vi "Main.vi"() -> ()   [LabVIEW 2020]
uses:
  Controls/Pages.ctl
  Controls/ManualTestParameters.ctl
  Controls/AutomaticalTestParameters.ctl
  <vilib>/express/express analysis/Spectral/Block/exnSpectralBlock spectral measurements power poly.vi
  <vilib>/express/express analysis/Spectral/Block/exnSpectralBlock spectral measurements power DDT.vi
  <vilib>/Utility/file.llb/Write Delimited Spreadsheet (string).vi
  <vilib>/express/express analysis/Spectral/XNode/ExpressSpectralMeasurementsBlockNode.xnode
panel:
  in  "Tab Control":T1=enum."自動測試/Automatical Test"
  in  "Manual Stop":bool
  in  "Manual Start":bool
  out "REVO. Alternate":dbl
  out "Manual Deflection":dbl
  out "BEND. Moment":dbl
  out "Tachometer":dbl
  in  "Order Open":bool
  in  "Auto Open":bool
  in  "Drive Up":bool
  in  "Drive Down":bool
  in  "Lamp On":bool
  in  "Lamp Off":bool
  out "Deflection":cluster{"probe x":dbl[], "probe y":dbl[]}[](graph)
  out "Power Spectrum":dynamicdata(graph)=[{"t0"=timestamp(0 s since 1904-01-01), "dt"=10.0, "Y"=[7.532951334960212e-36, 1.7210013073600366e-33, 2.9039505459542225e-32, 9.336804130865817e-32, 3.125000000000003, 12.499999999999991, 3.1249999999999942, 1.4832349234044934e-31, 1.9137290229811662e-32, 1.276010813808381e-32, 1.540768629947705e-33, 7.89098636152294e-33, 3.719445115484756e-33, 2.1300708903905205e-33, 4.0510738555792935e-32, 4.175831739872474e-32, 7.199150609282058e-32, 7.992518441924071e-34, 3.15189982829308e-33, 1.5483081913227212e-32, 1.6373277826284248e-32, 2.2138266275822093e-34, 4.406252635318449e-33, 3.438771975347449e-33, 1.3240311408006708e-32, 1.864729947416446e-31, 3.1076446481504366e-32, 1.351580401177905e-32, 1.0666709108251642e-32, 3.703047405966511e-33, 6.290037498430406e-32, 1.2794414884957584e-33, 3.841586151461403e-33, 7.984806335457992e-34, 3.5638767150319115e-32, 4.1301066800437274e-32, 4.0393850154926674e-32, 3.13032293215036e-33, 1.4282906971287278e-33, 3.758265447602662e-33, 1.0313371534831396e-31, 1.0624643515683048e-32, 4.981671705505977e-33, 1.9271055708889898e-33, 3.687743394522952e-32, 2.70478781889346e-31, 6.205033963623051e-32, 3.6208769442789164e-32, 9.98040293718275e-33, 2.859575628363253e-33], "attributes"=variant("NI_ChannelName"=variant(string "Sine (Power Spectrum)"), "NI_ExpIsRelativeTime"=variant(bool TRUE), "NI_ExpStartTimeStamp"=variant(timestamp timestamp(3762475107.3663697 s since 1904-01-01)), "NI_ExpTimeStamp"=variant(timestamp timestamp(3762475118.76637 s since 1904-01-01)), "NI_ExpXDimension"=variant(string "f"), "NI_OriginalChannelName"=variant(string "Sine"))}]
  in  "Reso Start":bool
  in  "Reso Stop":bool
  out "EstimatedTime_Value":dbl=290.99090337753296 format="%#_3g"
  in  "Auto Stop":bool
  out "Deflection_Value":dbl
  in  "Deflection_Setting":dbl=0.8
  out "Cycles_Value":dbl
  in  "Cycles_Setting":dbl=100.0
  out "BEND. Moment_Value":dbl
  in  "BEND. Moment_Setting":dbl=95.0
  out "Tachometer_Value":dbl
  in  "Tachometer_Setting":dbl=200.0
  out "Machine STA.":string="Running"
  in  "Auto Start":bool
  in  "Table":string[][](table)
  in  "Save Button":bool
  # "輪圈彎曲力矩耐久測試機"
  # "CORNERING BENDING ENDURANCE TESTER"
  # "金嵩盛機械股份有限公司承製"
  # "King Swen Sheng Machinery Co, Ltd."
  # "FAX: 886-3-4561597"
  # "TEL: 886-3-4384699"
  # "手動測試"
  # "Manual Test"
  # "迴轉轉速/Tachometer:"
  # "RPM"
  # "彎曲力矩/BEND. Moment:"
  # "N．m"
  # "負載偏移量/Deflection:"
  # "mm"
  # "主軸間距/REVO. Alternate:"
  # "M/M"
  # "共振測試"
  # "Resonance Test"
  # "自動測試"
  # "Automatical Test"
  # "機台狀況/Machine STA. :"
  # "設定值/Setting"
  # "實際值/Value"
  # "迴轉轉速/Tachometer:"
  # "RPM"
  # "力矩/BEND. Moment:"
  # "N．m"
  # "圈數/INT. Cycles:"
  # "圈"
  # "偏移量/Deflection:"
  # "mm"
  # "預計完成時間/Estimated Finish Time:"
  # "mins"
  # "報告產生"
  # "Report Generation"
  # "輪圈彎曲力矩耐久測試機"
  # "CORNERING BENDING ENDURANCE TESTER"
  # "金嵩盛機械股份有限公司承製"
  # "King Swen Sheng Machinery Co, Ltd."
  # "FAX: 886-3-4561597"
  # "TEL: 886-3-4384699"
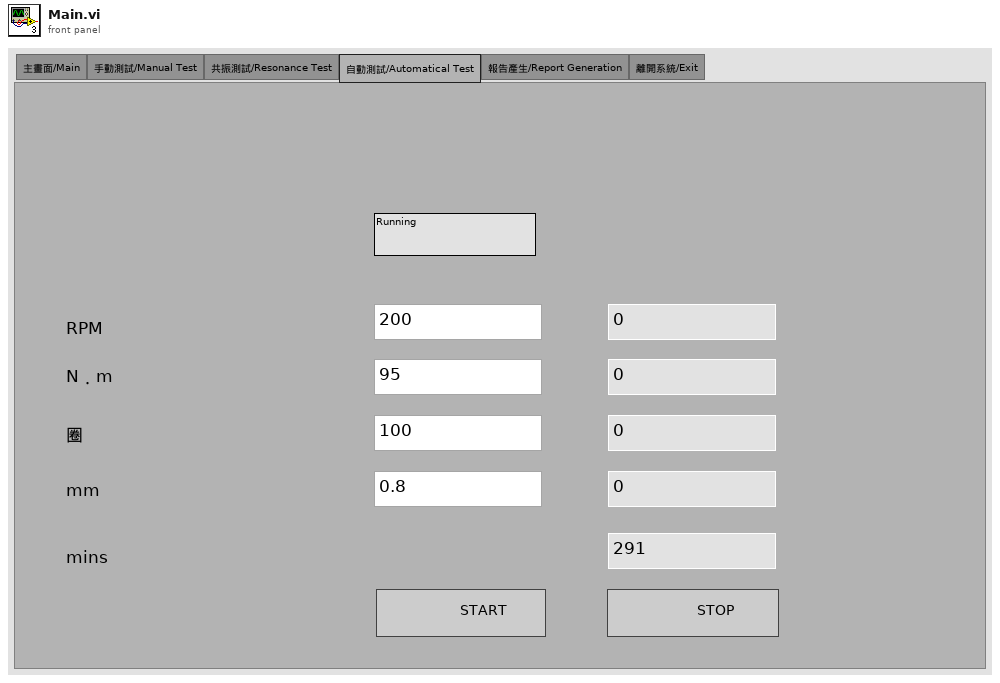
[diagram p1: front panel]
types:
  T1 = typedef "Pages.ctl" = enum32{"主畫面/Main", "手動測試/Manual Test", "共振測試/Resonance Test", "自動測試/Automatical Test", "報告產生/Report Generation", "離開系統/Exit"}
  T2 = typedef "AutomaticalTestParameters.ctl" = cluster{"Machine STA.":string, "Tachometer_Setting":dbl, "BEND. Moment_Setting":dbl, "Cycles_Setting":dbl, "Deflection_Setting":dbl, "Tachometer_Value":dbl, "BEND. Moment_Value":dbl, "Cycles_Value":dbl, "Deflection_Value":dbl, "EstimatedTime_Value":dbl, "Play Button":bool, "Stop Button":bool}
  T3 = typedef "ManualTestParameters.ctl" = cluster{"Order Open":bool, "Auto Open":bool, "Drive Up":bool, "Drive Down":bool, "Lamp On":bool, "Lamp Off":bool, "Tachometer":dbl, "BEND. Moment":dbl, "Deflection":dbl, "REVO. Alternate":dbl, "Drive Up Limit":dbl}
  T4 = enum8{"Enabled", "Disabled", "Disabled and Grayed Out"}
  T5 = cluster{"averaging mode":u16, "weighting mode":u16, "number of averages":u32}
  T6 = cluster{"dB On (F)":bool, "unwrap phase (F)":bool, "convert to degree (F)":bool}
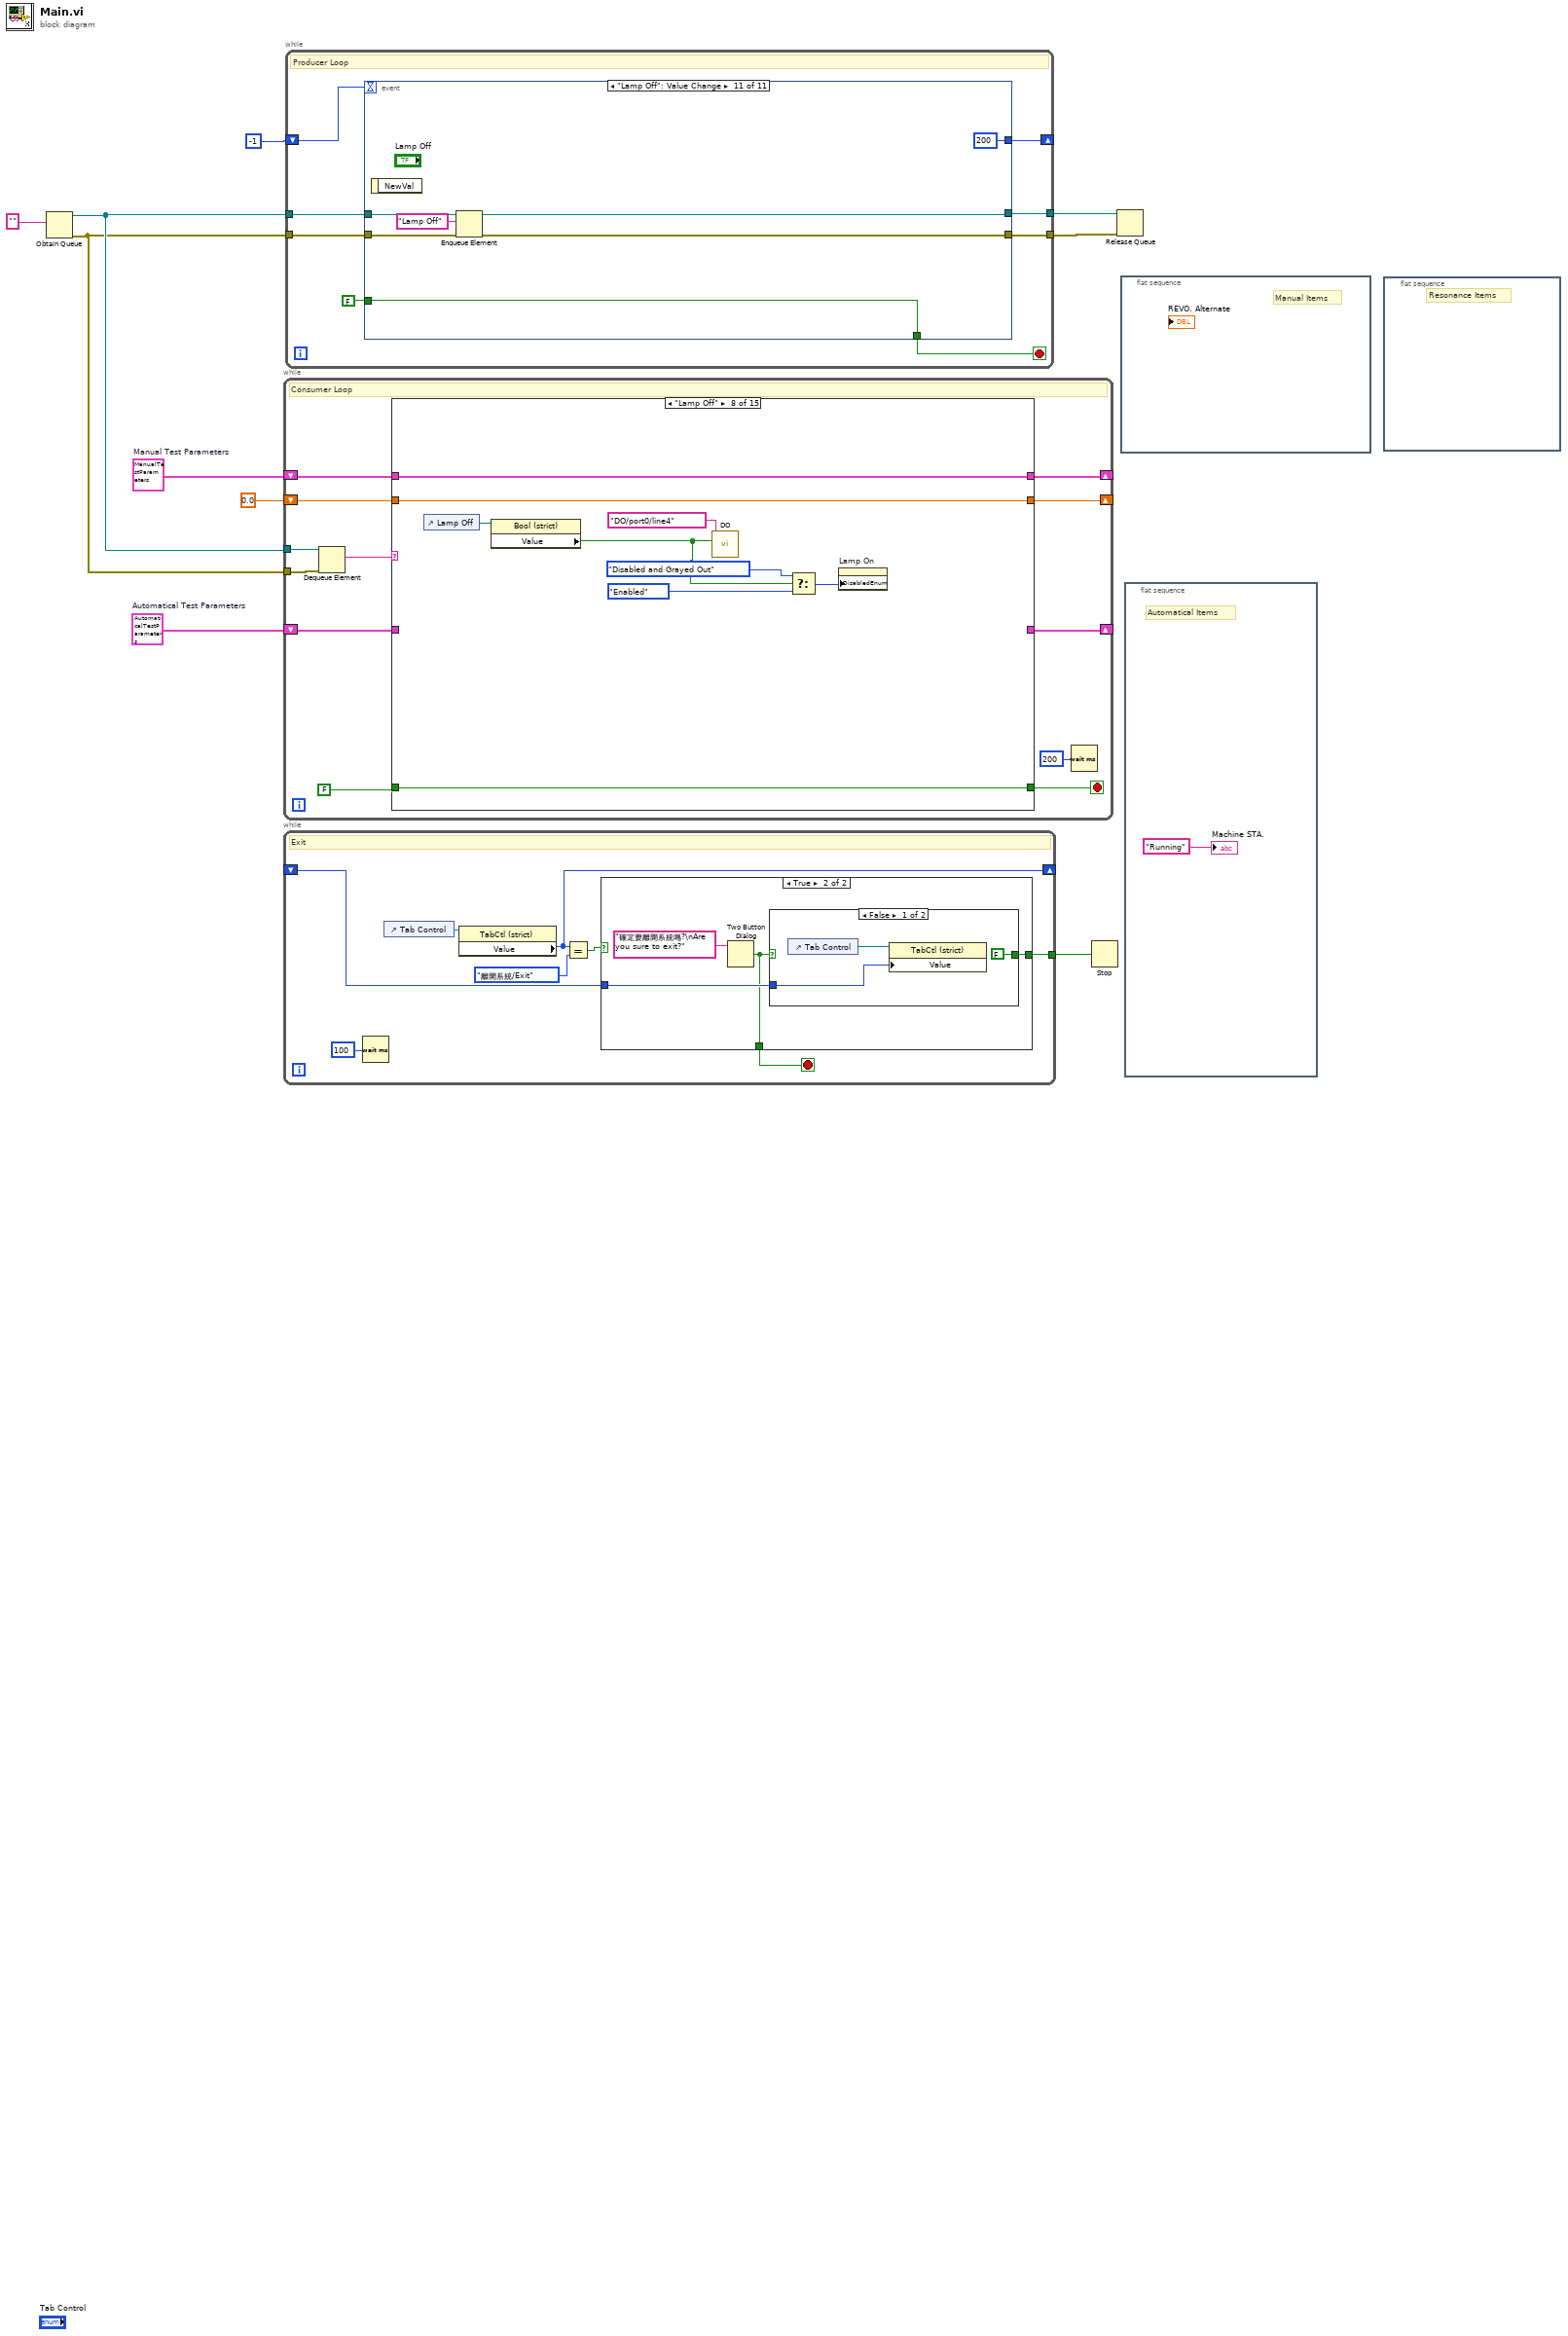
[diagram p0: block diagram]
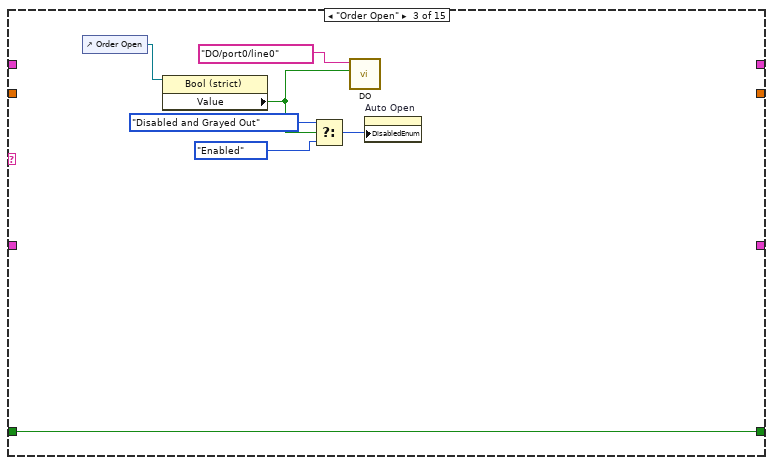
[diagram p4: hidden frame]
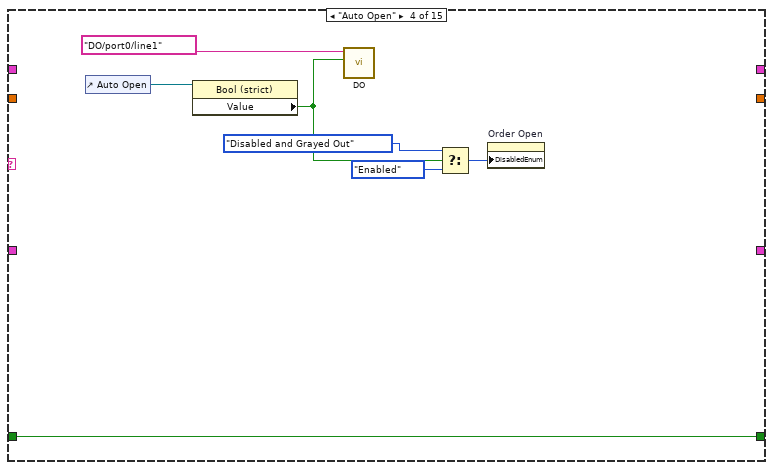
[diagram p5: hidden frame]
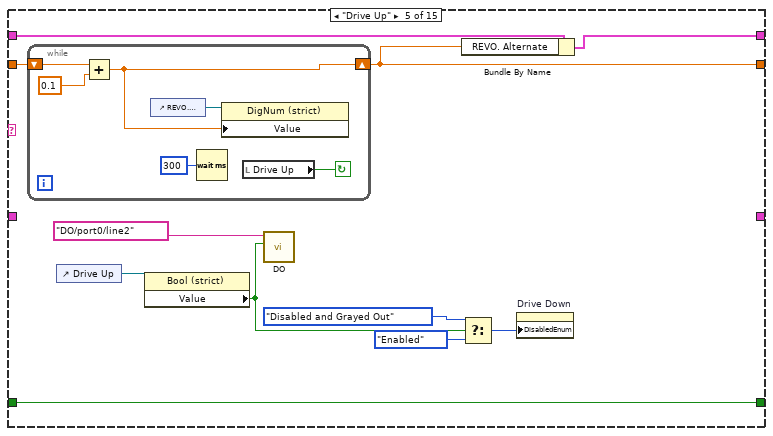
[diagram p6: hidden frame]
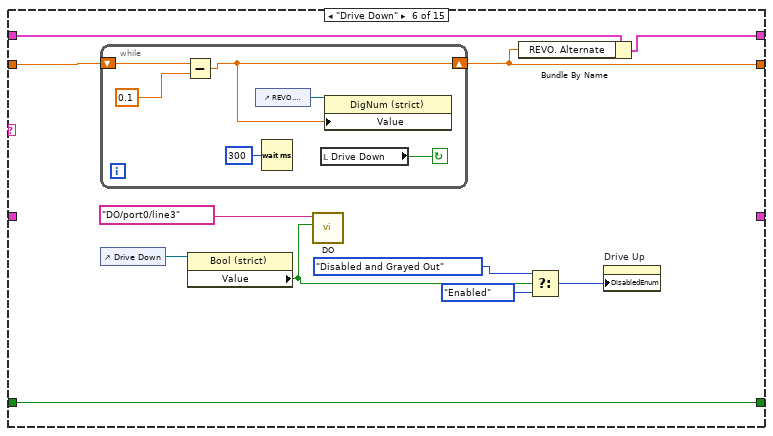
[diagram p7: hidden frame]
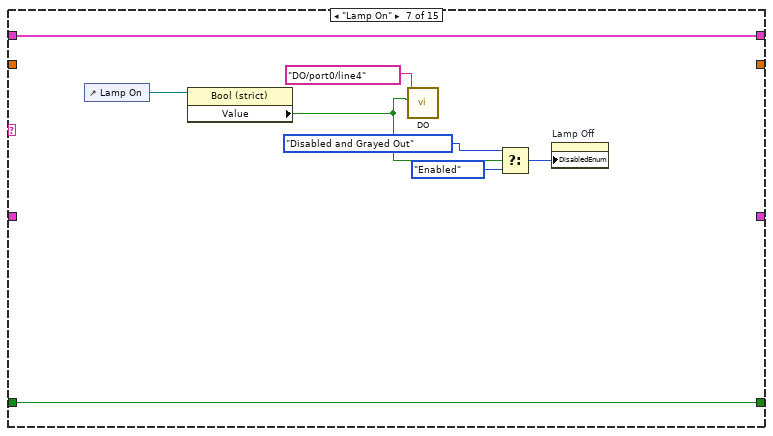
[diagram p8: hidden frame]
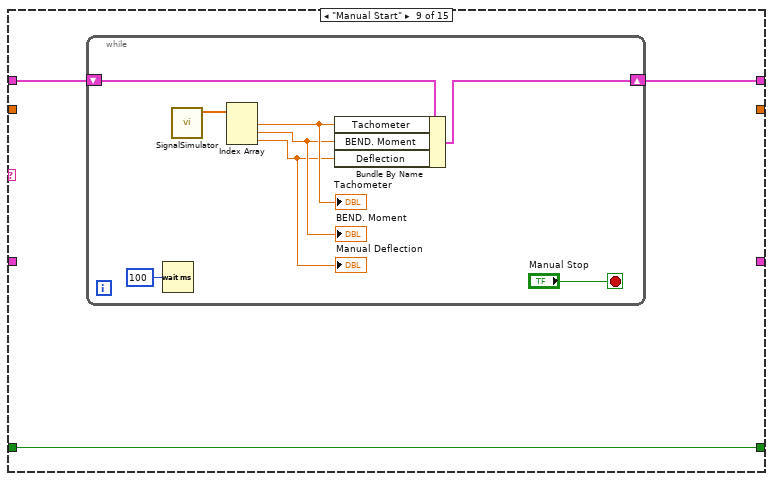
[diagram p9: hidden frame]
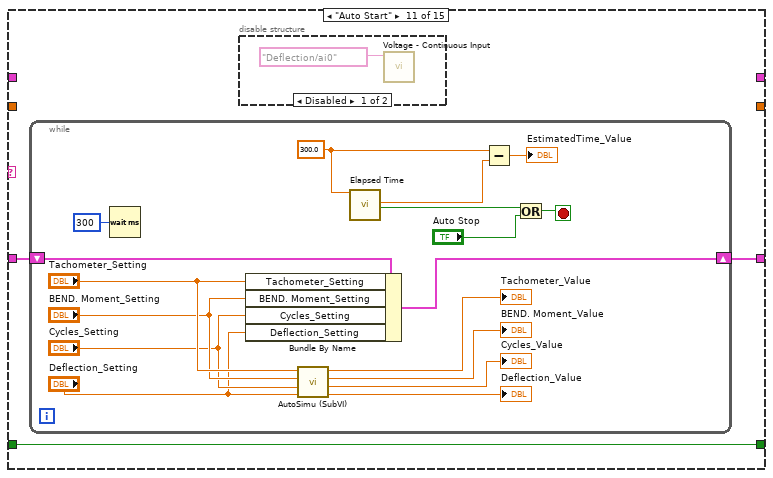
[diagram p11: hidden frame]
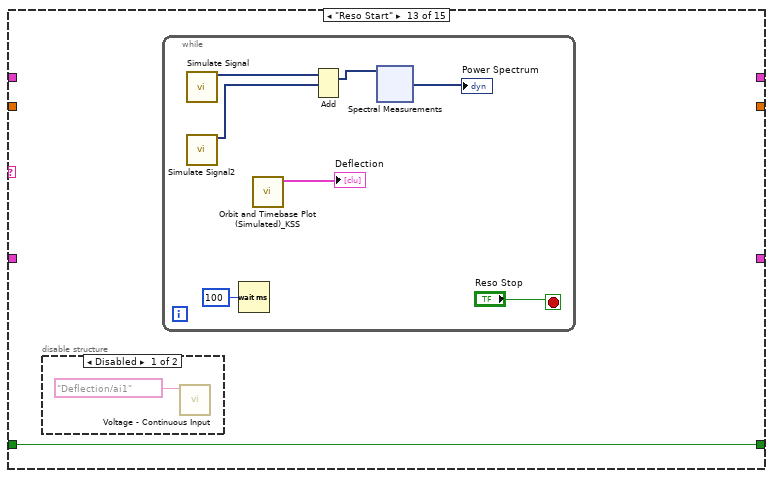
[diagram p14: hidden frame]
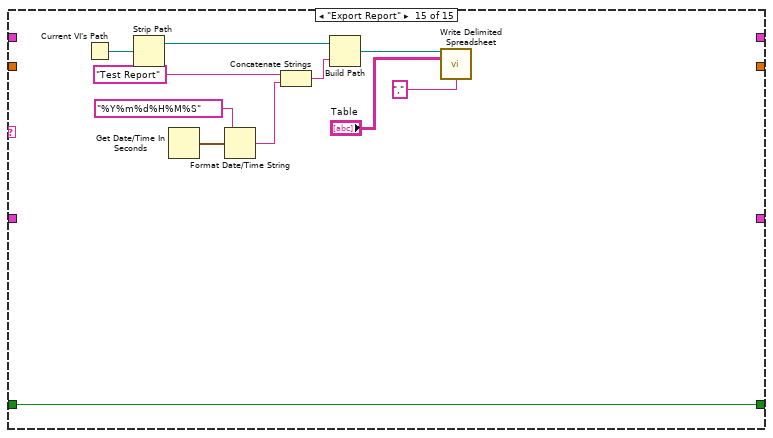
[diagram p17: hidden frame]
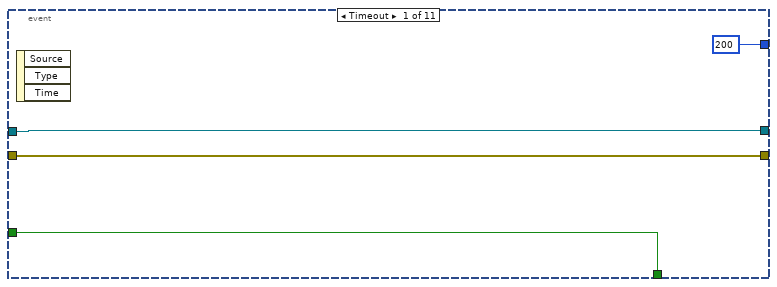
[diagram p18: hidden frame]
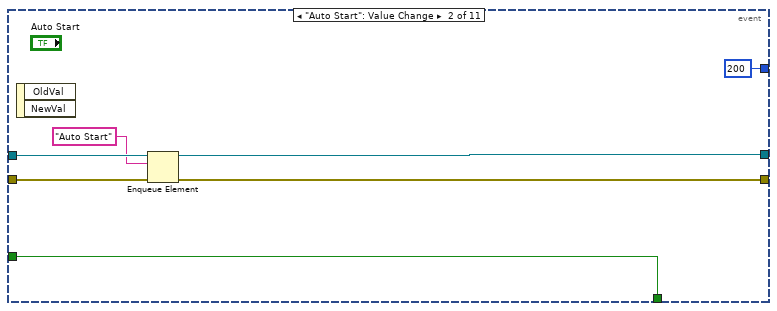
[diagram p19: hidden frame]
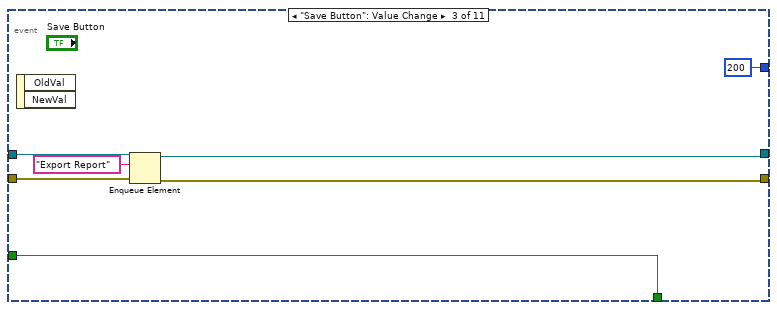
[diagram p20: hidden frame]
diagram:
  w1 = T2 {"Machine STA."="", "Tachometer_Setting"=0.0, "BEND. Moment_Setting"=0.0, "Cycles_Setting"=0.0, "Deflection_Setting"=0.0, "Tachometer_Value"=0.0, "BEND. Moment_Value"=0.0, "Cycles_Value"=0.0, "Deflection_Value"=0.0, "EstimatedTime_Value"=0.0, "Play Button"=FALSE, "Stop Button"=FALSE}  # Automatical Test Parameters
  w3 = T3 {"Order Open"=FALSE, "Auto Open"=FALSE, "Drive Up"=FALSE, "Drive Down"=FALSE, "Lamp On"=FALSE, "Lamp Off"=FALSE, "Tachometer"=0.0, "BEND. Moment"=0.0, "Deflection"=0.0, "REVO. Alternate"=0.0, "Drive Up Limit"=0.0}  # Manual Test Parameters
  n1 = Obtain Queue(element data type="") -> (queue out=w8:refnum<queue>, error out=w7:errorcluster)  [unwired: 4 in, 1 out]
  n2 = while {
    tunnel: w8 -> [w22]
    tunnel: w7 -> [w21]
    shift-right: [w16] -> _
    shift-left: w3 -> [w17]
    shift-right: [w14] -> _
    shift-left: 0.0 -> [w15]
    shift-right: [w11] -> _
    shift-left: w1 -> [w12]
    stop <- w19 stop-if-true
    # "Consumer Loop"
    n3 = Dequeue Element(queue=w22, error in (no error)=w21) -> (element=w20:string)  [unwired: 1 in, 3 out]
    n4 = case shown="\"Lamp Off\"" w20 {
      tunnel: [w23 w24 w31 w38 w49 w66 w80 w89 w92 w103 w106 w125 w126 w144 w155] -> w19
      tunnel: FALSE -> [w23 w24 w31 w38 w49 w66 w80 w89 w92 w103 w106 w125 w126 w144 w155]
      tunnel: w17 -> [_ _ _ _ w46 w63 w78 w87 w91 w102 _ _ _ _ _]
      tunnel: [_ _ _ _ w44 w62 w78 w87 w90 w102 _ _ _ _ _] -> w16
      tunnel: w15 -> [_ _ _ _ w45 w61 _ w86 _ w101 _ _ _ _ _]
      tunnel: [_ _ _ _ w43 w60 _ w86 _ w101 _ _ _ _ _] -> w14
      tunnel: w12 -> [_ _ _ _ _ _ _ _ _ _ w105 _ _ _ _]
      tunnel: [_ _ _ _ _ _ _ _ _ _ w104 _ _ _ _] -> w11
      frame "False", Default {
      }
      frame "-----Manual Test-----" {
      }
      frame "Order Open" {
        n5 = control-ref of="Order Open"() -> (w29:refnum<vi>)
        n6 = property class="Bool (strict)"(reference=w29) -> ("Value"=w28:bool)  [unwired: 1 in, 2 out]
        n7 = Select(t=T4."Disabled and Grayed Out", s=w28, f=T4."Enabled" ("Disabled")) -> (s? t:f=w25:T4)
        n8 = call "DO.vi"("data"=w28, "Line(s)"=tag "DO/port0/line0") -> ()  [unwired: 9 in, 1 out]
        n9 = property on="Auto Open" class="Bool (strict)"("DisabledEnum"=w25) -> ()  [unwired: 2 in, 2 out]
      }
      frame "Auto Open" {
        n10 = control-ref of="Auto Open"() -> (w36:refnum<vi>)
        n11 = property class="Bool (strict)"(reference=w36) -> ("Value"=w35:bool)  [unwired: 1 in, 2 out]
        n12 = call "DO.vi"("data"=w35, "Line(s)"=tag "DO/port0/line1") -> ()  [unwired: 9 in, 1 out]
        n13 = Select(t=T4."Disabled and Grayed Out" ("Disabled"), s=w35, f=T4."Enabled") -> (s? t:f=w32:T4)
        n14 = property on="Order Open" class="Bool (strict)"("DisabledEnum"=w32) -> ()  [unwired: 2 in, 2 out]
      }
      frame "Drive Up" {
        n15 = while {
          shift-right: [w50] -> w43
          shift-left: w45 -> [w55]
          stop <- w53 continue-if-true
          n16 = Add(x=w55, y=0.1) -> (x+y=w50:dbl)
          n17 = control-ref of="REVO. Alternate"() -> (w51:refnum<vi>)
          n18 = Wait (ms)(milliseconds to wait=u32 300) -> ()  [unwired: 1 out]
          n19 = property class="DigNum (strict)"(reference=w51, "Value"=w50) -> ()  [unwired: 1 in, 2 out]
          n20 = local read "Drive Up"() -> (w53:bool)
        }
        n21 = control-ref of="Drive Up"() -> (w47:refnum<vi>)
        n22 = property class="Bool (strict)"(reference=w47) -> ("Value"=w42:bool)  [unwired: 1 in, 2 out]
        n23 = call "DO.vi"("data"=w42, "Line(s)"=tag "DO/port0/line2") -> ()  [unwired: 9 in, 1 out]
        n24 = Bundle By Name(cluster=w46, "REVO. Alternate"=w43) -> (w44:T3)
        n25 = Select(t=T4."Disabled and Grayed Out" ("Disabled"), s=w42, f=T4."Enabled") -> (s? t:f=w39:T4)
        n26 = property on="Drive Down" class="Bool (strict)"("DisabledEnum"=w39) -> ()  [unwired: 2 in, 2 out]
      }
      frame "Drive Down" {
        n27 = while {
          shift-right: [w69] -> w60
          shift-left: w61 -> [w71]
          stop <- w68 continue-if-true
          n28 = Subtract(x=w71, y=0.1) -> (x-y=w69:dbl)
          n29 = control-ref of="REVO. Alternate"() -> (w70:refnum<vi>)
          n30 = Wait (ms)(milliseconds to wait=u32 300) -> ()  [unwired: 1 out]
          n31 = local read "Drive Down"() -> (w68:bool)
          n32 = property class="DigNum (strict)"(reference=w70, "Value"=w69) -> ()  [unwired: 1 in, 2 out]
        }
        n33 = control-ref of="Drive Down"() -> (w64:refnum<vi>)
        n34 = property class="Bool (strict)"(reference=w64) -> ("Value"=w57:bool)  [unwired: 1 in, 2 out]
        n35 = call "DO.vi"("data"=w57, "Line(s)"=tag "DO/port0/line3") -> ()  [unwired: 9 in, 1 out]
        n36 = Bundle By Name(cluster=w63, "REVO. Alternate"=w60) -> (w62:T3)
        n37 = Select(t=T4."Disabled and Grayed Out" ("Disabled"), s=w57, f=T4."Enabled") -> (s? t:f=w56:T4)
        n38 = property on="Drive Up" class="Bool (strict)"("DisabledEnum"=w56) -> ()  [unwired: 2 in, 2 out]
      }
      frame "Lamp On" {
        n39 = control-ref of="Lamp On"() -> (w74:refnum<vi>)
        n40 = property class="Bool (strict)"(reference=w74) -> ("Value"=w73:bool)  [unwired: 1 in, 2 out]
        n41 = call "DO.vi"("data"=w73, "Line(s)"=tag "DO/port0/line4") -> ()  [unwired: 9 in, 1 out]
        n42 = Select(t=T4."Disabled and Grayed Out" ("Disabled"), s=w73, f=T4."Enabled") -> (s? t:f=w75:T4)
        n43 = property on="Lamp Off" class="Bool (strict)"("DisabledEnum"=w75) -> ()  [unwired: 2 in, 2 out]
      }
      frame "Lamp Off" {
        n44 = control-ref of="Lamp Off"() -> (w82:refnum<vi>)
        n45 = property class="Bool (strict)"(reference=w82) -> ("Value"=w81:bool)  [unwired: 1 in, 2 out]
        n46 = call "DO.vi"("data"=w81, "Line(s)"=tag "DO/port0/line4") -> ()  [unwired: 9 in, 1 out]
        n47 = Select(t=T4."Disabled and Grayed Out" ("Disabled"), s=w81, f=T4."Enabled") -> (s? t:f=w83:T4)
        n48 = property on="Lamp On" class="Bool (strict)"("DisabledEnum"=w83) -> ()  [unwired: 2 in, 2 out]
      }
      frame "Manual Start" {
        n49 = while {
          shift-right: [w96] -> w90
          shift-left: w91 -> [w98]
          stop <- "Manual Stop" stop-if-true
          n50 = Wait (ms)(milliseconds to wait=u32 100) -> ()  [unwired: 1 out]
          n51 = call "SignalSimulator.vi"() -> ("Array"=w100:dbl[])  [unwired: 11 in]
          n52 = Index Array(array=w100) -> (element #1=w95:dbl, element #2=w94:dbl, element #3=w93:dbl)  [unwired: 3 in]
          "Tachometer" <- w95
          "BEND. Moment" <- w94
          "Manual Deflection" <- w93
          n53 = Bundle By Name(cluster=w98, "Tachometer"=w95, "BEND. Moment"=w94, "Deflection"=w93) -> (w96:T3)
        }
      }
      frame "-----Automatical Test-----" {
      }
      frame "Auto Start" {
        n54 = while {
          shift-right: [w123] -> w104
          shift-left: w105 -> [w124]
          stop <- w113 stop-if-true
          w112 = 300.0 ("Time Target (s)")
          n55 = Wait (ms)(milliseconds to wait=u32 300) -> ()  [unwired: 1 out]
          n56 = Bundle By Name(cluster=w124, "Tachometer_Setting"="Tachometer_Setting", "BEND. Moment_Setting"="BEND. Moment_Setting", "Cycles_Setting"="Cycles_Setting", "Deflection_Setting"="Deflection_Setting") -> (w123:T2)
          n57 = call "AutoSimu (SubVI).vi"("Deflection_Setting 5"="Deflection_Setting", "Cycles_Setting"="Cycles_Setting", "BEND. Moment_Setting"="BEND. Moment_Setting", "Tachometer_Setting"="Tachometer_Setting") -> ("Deflection_Setting"=→"Deflection_Value":dbl, "Deflection_Setting 2"=→"Cycles_Value":dbl, "Deflection_Setting 3"=→"BEND. Moment_Value":dbl, "Deflection_Setting 4"=→"Tachometer_Value":dbl)  [unwired: 4 in]
          n58 = call "Elapsed Time"("Time Target (s)"=w112) -> ("Elapsed Time (s)"=w111:dbl, "Time has Elapsed"=w115:bool)  [unwired: 11 in, 6 out]
          n59 = Subtract(x=w112, y=w111) -> (x-y=→"EstimatedTime_Value":dbl)
          n60 = Or(x=w115, y="Auto Stop") -> (x .or. y?=w113:bool)
        }
        n61 = disable-structure shown="Disabled" {
          frame Disabled {
            n62 = call "Voltage - Continuous Input.vi"("Physical Channel"=tag "Deflection/ai0") -> ()  [unwired: 9 in, 2 out]
          }
          frame Enabled {
          }
        }
      }
      frame "-----Resonance Test-----" {
      }
      frame "Reso Start" {
        n63 = disable-structure shown="Disabled" {
          frame Disabled {
            n64 = call "Voltage - Continuous Input.vi"("Physical Channel"=tag "Deflection/ai1") -> ()  [unwired: 9 in, 2 out]
          }
          frame Enabled {
          }
        }
        n65 = while {
          stop <- "Reso Stop" stop-if-true
          n66 = call "Simulate Signal"() -> ("Sine"=w129:dynamicdata)  [unwired: 14 in, 1 out]
          n67 = call "Simulate Signal2"() -> ("Sine"=w128:dynamicdata)  [unwired: 14 in, 1 out]
          n68 = Wait (ms)(milliseconds to wait=u32 100) -> ()  [unwired: 1 out]
          n69 = call "Orbit and Timebase Plot (Simulated)_KSS.vi"() -> ("XY Graph"=→"Deflection":cluster{"probe x":dbl[], "probe y":dbl[]}[])  [unwired: 10 in, 1 out]
          n70 = Add(1:w128, 2:w129) -> (0:w127:dynamicdata)  [unwired: 1 in, 1 out]
          n71 = xnode "Spectral Measurements"("Signals"=w127) -> ("Power Spectrum"=→"Power Spectrum":dynamicdata)  [unwired: 1 in, 1 out]
        }
      }
      frame "-----Report Generation-----" {
      }
      frame "Export Report" {
        n72 = Current VI's Path() -> (path=w153:path)
        n73 = Strip Path(path=w153) -> (stripped path=w151:path)  [unwired: 1 out]
        n74 = Get Date/Time In Seconds() -> (seconds since 1Jan1904=w150:timestamp)
        n75 = Format Date/Time String(time format string (%c)="%Y%m%d%H%M%S", seconds (now)=w150) -> (date/time string=w146:string)  [unwired: 1 in]
        n76 = Concatenate Strings("Test Report" ("string"), w146) -> (w148:string)
        n77 = Build Path(base path=w151, name or relative path=w148) -> (appended path=w152:path)
        n78 = call-poly <vilib>:"Write Delimited Spreadsheet.vi"("file path (dialog if empty)"=w152, "2D data"="Table", "delimiter (\\t)"="," ("delimiter (\\t)")) -> ()  [unwired: 11 in, 2 out]
      }
    }
    n79 = Wait (ms)(milliseconds to wait=u32 200) -> ()  [unwired: 1 out]
  }
  n80 = while {
    tunnel: [w160] -> w10
    shift-right: [w159] -> _
    shift-left: _ -> [w158]
    stop <- w157 stop-if-true
    # "Exit"
    n81 = Wait (ms)(milliseconds to wait=u32 100) -> ()  [unwired: 1 out]
    n82 = control-ref of="Tab Control"() -> (w163:refnum<vi>)
    n83 = property class="TabCtl (strict)"(reference=w163) -> ("Value"=w159:T1)  [unwired: 1 in, 2 out]
    n84 = Equal?(x=w159, y=Pages."離開系統/Exit") -> (x = y?=w161:bool)
    n85 = case shown="True" w161 {
      tunnel: [FALSE w168] -> w160
      tunnel: w158 -> [_ w167]
      tunnel: [FALSE ("T button?") w166] -> w157
      frame False {
      }
      frame True {
        n86 = Two Button Dialog(message="確定要離開系統嗎?\nAre you sure to exit?") -> (T button?=w166:bool)  [unwired: 2 in]
        n87 = case shown="False" w166 {
          selector: w166 -> [_ w173]
          tunnel: [FALSE w173] -> w168
          tunnel: w167 -> [w170 _]
          frame False {
            n88 = control-ref of="Tab Control"() -> (w172:refnum<vi>)
            n89 = property class="TabCtl (strict)"(reference=w172, "Value"=w170) -> ()  [unwired: 1 in, 2 out]
          }
          frame True {
          }
        }
      }
    }
  }
  n90 = while {
    tunnel: w8 -> [w181]
    tunnel: w7 -> [w180]
    tunnel: [w179] -> w6
    tunnel: [w178] -> w5
    shift-right: [w175] -> _
    shift-left: -1 -> [w174]
    stop <- w177 stop-if-true
    # "Producer Loop"
    n91 = event shown="[10] \"Lamp Off\": Value Change" {
      selector: _ -> [_ _ _ _ _ _ _ _ _ _ _]
      dyn-events: _ -> [_ _ _ _ _ _ _ _ _ _ _]
      timeout: w174 -> [_ _ _ _ _ _ _ _ _ _ _]
      tunnel: w181 -> [w185 w192 w199 w206 w213 w220 w227 w234 w241 w248 w255]
      tunnel: w180 -> [w184 w191 w198 w205 w212 w219 w226 w233 w240 w247 w254]
      tunnel: [w185 w190 w197 w204 w210 w216 w224 w232 w238 w245 w252] -> w179
      tunnel: [w184 w189 w196 w203 w209 w215 w223 w231 w237 w244 w251] -> w178
      tunnel: [w183 w186 w193 w200 w208 w218 w222 w229 w236 w243 w250] -> w177
      tunnel: FALSE -> [w183 w186 w193 w200 w208 w218 w222 w229 w236 w243 w250]
      tunnel: [200 200 200 200 200 200 200 200 200 200 200] -> w175
      event Timeout {
        n92 = event-data() -> ()  [unwired: 1 in, 3 out]
      }
      event "Auto Start": Value Change {
        n93 = event-data() -> ()  [unwired: 1 in, 2 out]
        n94 = Enqueue Element(queue=w192, element="Auto Start", error in (no error)=w191) -> (queue out=w190:refnum<queue>, error out=w189:errorcluster)  [unwired: 1 in, 1 out]
      }
      event "Save Button": Value Change {
        n95 = event-data() -> ()  [unwired: 1 in, 2 out]
        n96 = Enqueue Element(queue=w199, element="Export Report", error in (no error)=w198) -> (queue out=w197:refnum<queue>, error out=w196:errorcluster)  [unwired: 1 in, 1 out]
      }
      event "Reso Start": Value Change {
        n97 = event-data() -> ()  [unwired: 1 in, 2 out]
        n98 = Enqueue Element(queue=w206, element="Reso Start", error in (no error)=w205) -> (queue out=w204:refnum<queue>, error out=w203:errorcluster)  [unwired: 1 in, 1 out]
      }
      event "Order Open": Value Change {
        n99 = event-data() -> ()  [unwired: 1 in, 1 out]
        n100 = Enqueue Element(queue=w213, element="Order Open", error in (no error)=w212) -> (queue out=w210:refnum<queue>, error out=w209:errorcluster)  [unwired: 1 in, 1 out]
      }
      event "Manual Start": Value Change {
        n101 = event-data() -> ()  [unwired: 1 in, 1 out]
        n102 = Enqueue Element(queue=w220, element="Manual Start", error in (no error)=w219) -> (queue out=w216:refnum<queue>, error out=w215:errorcluster)  [unwired: 1 in, 1 out]
      }
      event "Auto Open": Value Change {
        n103 = event-data() -> ()  [unwired: 1 in, 1 out]
        n104 = Enqueue Element(queue=w227, element="Auto Open", error in (no error)=w226) -> (queue out=w224:refnum<queue>, error out=w223:errorcluster)  [unwired: 1 in, 1 out]
      }
      event "Drive Up": Value Change {
        n105 = event-data() -> ()  [unwired: 1 in, 1 out]
        n106 = Enqueue Element(queue=w234, element="Drive Up", error in (no error)=w233) -> (queue out=w232:refnum<queue>, error out=w231:errorcluster)  [unwired: 1 in, 1 out]
      }
      event "Drive Down": Value Change {
        n107 = event-data() -> ()  [unwired: 1 in, 1 out]
        n108 = Enqueue Element(queue=w241, element="Drive Down", error in (no error)=w240) -> (queue out=w238:refnum<queue>, error out=w237:errorcluster)  [unwired: 1 in, 1 out]
      }
      event "Lamp On": Value Change {
        n109 = event-data() -> ()  [unwired: 1 in, 1 out]
        n110 = Enqueue Element(queue=w248, element="Lamp On", error in (no error)=w247) -> (queue out=w245:refnum<queue>, error out=w244:errorcluster)  [unwired: 1 in, 1 out]
      }
      event "Lamp Off": Value Change {
        n111 = event-data() -> ()  [unwired: 1 in, 1 out]
        n112 = Enqueue Element(queue=w255, element="Lamp Off", error in (no error)=w254) -> (queue out=w252:refnum<queue>, error out=w251:errorcluster)  [unwired: 1 in, 1 out]
      }
    }
  }
  n113 = Stop(stop? (T)=w10) -> ()
  n114 = Release Queue(queue=w6, error in (no error)=w5) -> ()  [unwired: 1 in, 3 out]
  n115 = flat-sequence {
    frame #0 {
      # "Manual Items"
    }
  }
  n116 = flat-sequence {
    frame #0 {
      # "Automatical Items"
      "Machine STA." <- "Running" ("Machine STA.")
    }
  }
  n117 = flat-sequence {
    frame #0 {
      # "Resonance Items"
    }
  }
